vi "main-light-switch.vi"(7 "LabVIEW Web Service Request":refnum<class "Web Request.lvclass">, 11 "state":bool) -> (3 "state-response":bool)   [LabVIEW 2023]
uses:
  <vilib>/wsapi/Web Request.lvclass
  Actuators.vi
panel:
  # "INPUT"
  # "OUTPUT"
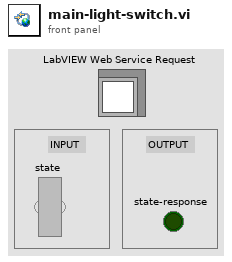
[diagram p1: front panel]
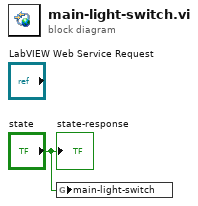
[diagram p0: block diagram]
diagram:
  n1 = global write "Actuators.vi" "main-light-switch"("state") -> ()
  "state-response" <- "state"
